vi "main.vi"() -> ()   [LabVIEW 2019, in "RT_Game.lvlib"]
uses:
  RT_Game.lvlib
  Globals.vi
  <vilib>/Utility/error.llb/Error Cluster From Error Code.vi
  <vilib>/ErrorRing/Error Ring.xnode
  Engine/Engine.lvclass
  <vilib>/NI_Real-Time Target Support.lvlib
panel:
  in  "SimulateError":bool
  out "delta t":dbl(graph)=11.0
  out "cpu":cluster{"Total (%)":dbl, "Total (%)":dbl}(graph)={"Total (%)"=36.40655155071103, "Total (%)"=28.773757553198372}
  in  "Stop":bool
  out "Error Out":errorcluster
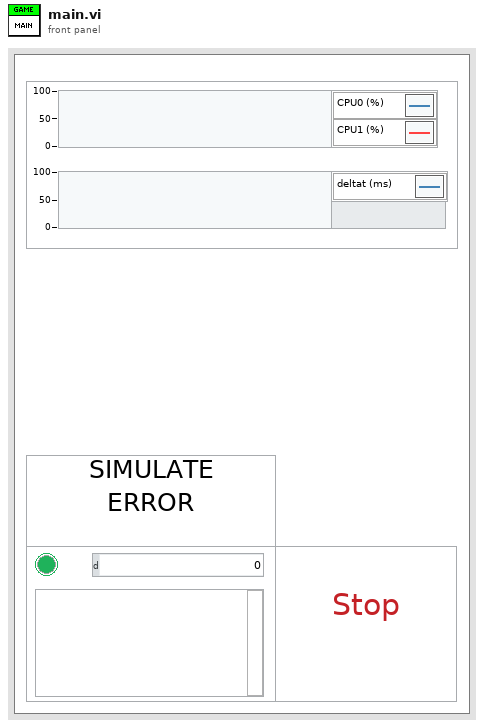
[diagram p1: front panel]
types:
  T1 = typedef "NI_Real-Time Target Support.lvlib/RT CPU Load.ctl" = cluster{"Total (%)":dbl, "Time Critical (%)":dbl, "Timed Structures (%)":dbl, "High (%)":dbl, "Above Normal (%)":dbl, "Normal (%)":dbl, "Background (%)":dbl, "Idle (%)":dbl, "ISR (%)":dbl}
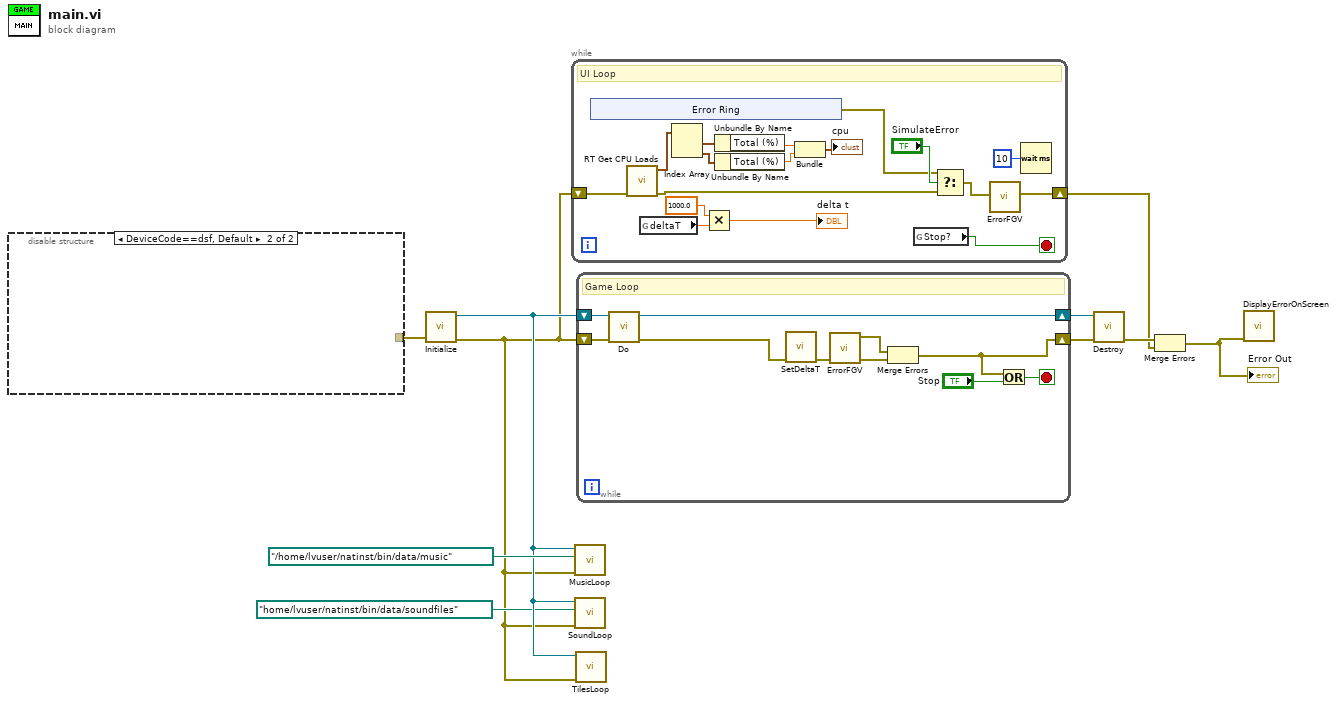
[diagram p0: block diagram]
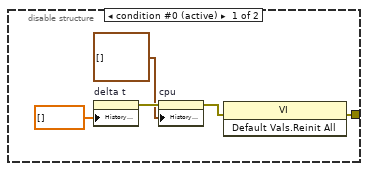
[diagram p2: hidden frame]
diagram:
  n1 = disable-structure shown="DeviceCode==dsf, Default" {
    disable-tunnel: [w15 _] -> w5
    frame condition #0 (active) {
      n2 = property on="delta t" class="WFChart (strict)"("History Data"=dbl[] []) -> (error out=w13:errorcluster)  [unwired: 2 in, 1 out]
      n3 = property on="cpu" class="WFChart (strict)"(error in=w13, "History Data"=cluster{"Total (%)":dbl, "Total (%)":dbl}[] []) -> (error out=w14:errorcluster)  [unwired: 1 in, 1 out]
      n4 = invoke class="VI" method="Default Vals.Reinit All"(error in=w14) -> (error out=w15:errorcluster)  [unwired: 2 in, 2 out]
    }
    frame condition #1 {
    }
  }
  n5 = call "Initialize.vi"("error in (no error)"=w5) -> ("error out"=w3:errorcluster, "Engine out"=w7:refnum<class "Engine.lvclass">)  [unwired: 9 in]
  n6 = while {
    shift-right: [w24] -> w1
    shift-left: w3 -> [w25]
    stop <- w27 stop-if-true
    # "UI Loop"
    n7 = xnode "Error Ring"() -> ("error out"=w16:errorcluster)
    n8 = call <vilib>:"RT Get CPU Loads.vi"("error in (no error)"=w25) -> ("error out"=w18:errorcluster, "CPU loads"=w29:T1[])  [unwired: 9 in]
    n9 = global read "Globals.vi" "deltaT"() -> (w32:dbl)
    n10 = Index Array(array=w29) -> (element #1=w30:T1, element #2=w31:T1)  [unwired: 2 in]
    n11 = Multiply(x=1000.0, y=w32) -> (x*y=→"delta t":dbl)
    n12 = Unbundle By Name(w30) -> ("Total (%)"=w23:dbl)
    n13 = Unbundle By Name(w31) -> ("Total (%)"=w22:dbl)
    n14 = Bundle("Total (%)"=w23, "Total (%)"=w22) -> (→"cpu":cluster{"Total (%)":dbl, "Total (%)":dbl})  [unwired: 1 in]
    n15 = global read "Globals.vi" "Stop?"() -> (w27:bool)
    n16 = Select(t=w16, s="SimulateError", f=w18) -> (s? t:f=w19:errorcluster)
    n17 = call "ErrorFGV.vi"("error in (no error)"=w19) -> ("error out"=w24:errorcluster)  [unwired: 9 in, 1 out]
    n18 = Wait (ms)(milliseconds to wait=u32 10) -> ()  [unwired: 1 out]
  }
  n19 = call "MusicLoop.vi"("error in (no error)"=w3, "Tracks"=path "//home/lvuser/natinst/bin/data/music", "Engine in"=w7) -> ()  [unwired: 8 in, 1 out]
  n20 = call "SoundLoop.vi"("error in (no error)"=w3, "SoundsFolder"=path "/home/lvuser/natinst/bin/data/soundfiles", "Engine in"=w7) -> ()  [unwired: 8 in, 1 out]
  n21 = call "TilesLoop.vi"("error in (no error)"=w3, "Engine in"=w7) -> ()  [unwired: 9 in, 1 out]
  n22 = while {
    shift-right: [w41] -> w10
    shift-left: w7 -> [w46]
    shift-right: [w39] -> w9
    shift-left: w3 -> [w45]
    stop <- w43 stop-if-true
    # "Game Loop"
    n23 = call "Do.vi"("error in (no error)"=w45, "Engine in"=w46) -> ("error out"=w44:errorcluster, "Engine out"=w41:refnum<class "Engine.lvclass">)  [unwired: 8 in]
    n24 = call "SetDeltaT.vi"("error in (no error)"=w44) -> ("error out"=w42:errorcluster)  [unwired: 10 in]
    n25 = call "ErrorFGV.vi"() -> ("SlaveLoopError"=w38:errorcluster)  [unwired: 10 in, 1 out]
    n26 = Merge Errors(w38, w42) -> (w39:errorcluster)
    n27 = Or(x=w39, y="Stop") -> (x .or. y?=w43:bool)
  }
  n28 = call "Destroy.vi"("error in (no error)"=w9, "Engine in"=w10) -> ("error out"=w4:errorcluster)  [unwired: 9 in]
  n29 = Merge Errors(w4, w1) -> (w2:errorcluster)
  "Error Out" <- w2
  n30 = call "DisplayErrorOnScreen.vi"("error in (no error)"=w2) -> ()  [unwired: 11 in]
